vi "DSF.Engine.Plugin.Shutdown.vi"(8 "error in (no error)":errorcluster, 11 "Plugin in":refnum<class "DSF.Engine.Plugin.lvclass">) -> (0 "error out":errorcluster, 3 "Plugin out":refnum<class "DSF.Engine.Plugin.lvclass">)   [LabVIEW 2017, in "DSF.Engine.lvlib" / "DSF.Engine.Plugin.lvclass"]
uses:
  DSF.Engine.Plugin.lvclass
  DSF.Engine.Plugin.lvclass/DSF.Engine.Plugin.ctl
  Transceiver/DSF.Engine.Transceiver Thread.lvclass
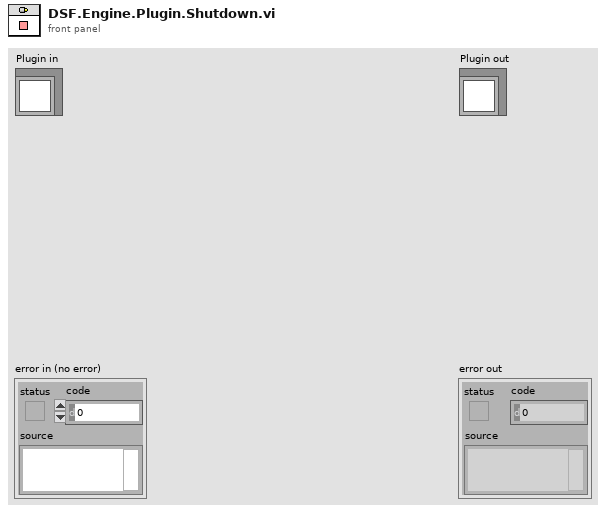
[diagram p1: front panel]
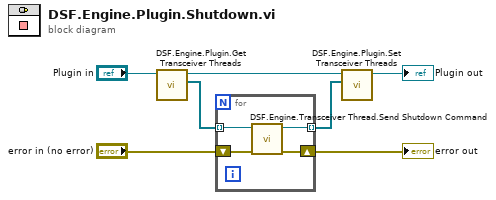
[diagram p0: block diagram]
diagram:
  n1 = call "DSF.Engine.Plugin.Get Transceiver Threads.vi"("Plugin in"="Plugin in") -> ("Transceiver Threads"=w3:refnum<class "DSF.Engine.Transceiver Thread.lvclass">[], "Plugin out"=w6:refnum<class "DSF.Engine.Plugin.lvclass">)  [unwired: 9 in]
  n2 = for {
    shift-right: [w8] -> w1
    shift-left: "error in (no error)" -> [w9]
    tunnel: [w10] -> w4 mode=indexing
    tunnel: w3 -> [w11] mode=indexing
    n3 = call "DSF.Engine.Transceiver Thread.Send Shutdown Command.vi"("error in (no error)"=w9, "Transceiver Thread in"=w11) -> ("error out"=w8:errorcluster, "Transceiver Thread out"=w10:refnum<class "DSF.Engine.Transceiver Thread.lvclass">)  [unwired: 8 in]
  }
  "error out" <- w1
  n4 = call "DSF.Engine.Plugin.Set Transceiver Threads.vi"("Transceiver Threads"=w4, "Plugin in"=w6) -> ("Plugin out"=→"Plugin out":refnum<class "DSF.Engine.Plugin.lvclass">)  [unwired: 9 in]
